vi "write_to_console.vi"(8 "error in":errorcluster, 11 "input_str":string) -> (0 "error out":errorcluster, 3 "res_str":string)   [LabVIEW 2021]
uses:
  console.vi
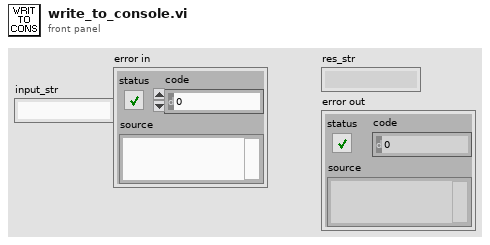
[diagram p1: front panel]
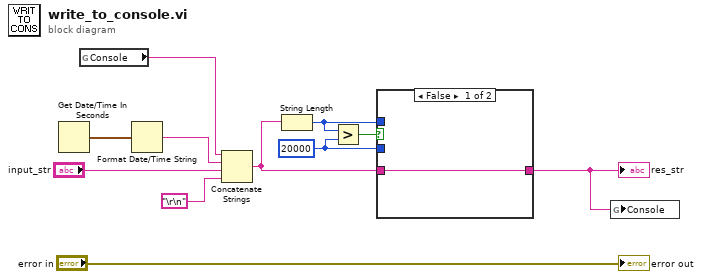
[diagram p0: block diagram]
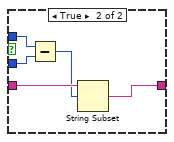
[diagram p2: hidden frame]
diagram:
  w6 = 20000 ("y")
  n1 = Get Date/Time In Seconds() -> (seconds since 1Jan1904=w4:timestamp)
  n2 = global read "console.vi" "Console"() -> (w2:string)
  n3 = Format Date/Time String(seconds (now)=w4) -> (date/time string=w3:string)  [unwired: 2 in]
  n4 = Concatenate Strings(w2, w3, "input_str", "\r\n") -> (w8:string)
  n5 = String Length(string=w8) -> (length=w7:i32)
  n6 = Greater?(x=w7, y=w6) -> (0:w9:bool)
  n7 = case shown="False" w9 {
    tunnel: w8 -> [w12 w17]
    tunnel: w7 -> [_ w16]
    tunnel: w6 -> [_ w15]
    tunnel: [w12 w13] -> w5
    frame False {
    }
    frame True {
      n8 = Subtract(x=w16, y=w15) -> (x-y=w14:i32)
      n9 = String Subset(string=w17, offset (0)=w14) -> (substring=w13:string)  [unwired: 1 in]
    }
  }
  "res_str" <- w5
  n10 = global write "console.vi" "Console"(w5) -> ()
  "error out" <- "error in"
